vi "Enum Symbol to String.vi"(10 "Symbol Enum In":T1) -> (2 "Symbol String Out":string)   [LabVIEW 2013]
uses:
  enum_Symbols.ctl
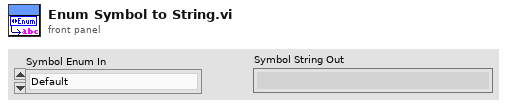
[diagram p1: front panel]
types:
  T1 = typedef "enum_Symbols.ctl" = enum16{"Default", "Analog Input", "Analog Output", "Digital Input", "Digital Output", "PWM Input", "PWM Output"}
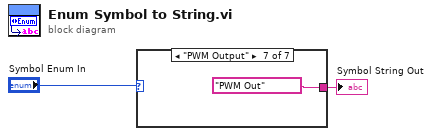
[diagram p0: block diagram]
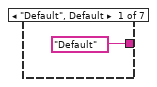
[diagram p2: hidden frame]
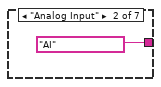
[diagram p3: hidden frame]
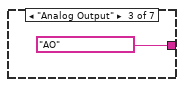
[diagram p4: hidden frame]
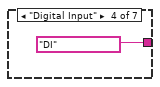
[diagram p5: hidden frame]
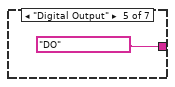
[diagram p6: hidden frame]
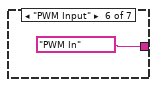
[diagram p7: hidden frame]
diagram:
  n1 = case shown="\"PWM Output\"" "Symbol Enum In" {
    tunnel: ["Default" ("Symbol 2") "AI" ("Symbol 2") "AO" ("Symbol 2") "DI" ("Symbol 2") "DO" ("Symbol 2") "PWM In" ("Symbol 2") "PWM Out" ("Symbol 2")] -> w1
    frame "Default", Default {
    }
    frame "Analog Input" {
    }
    frame "Analog Output" {
    }
    frame "Digital Input" {
    }
    frame "Digital Output" {
    }
    frame "PWM Input" {
    }
    frame "PWM Output" {
    }
  }
  "Symbol String Out" <- w1
